vi "时间日期字符串转时间数组.vi"(11 "日期/时间字符串":string) -> (3 "时间数组":i32[](array[numeric]))   [LabVIEW 2016, in "TimingControl.lvlib" / "TimingControl.lvclass"]
uses:
  TimingControl.lvclass
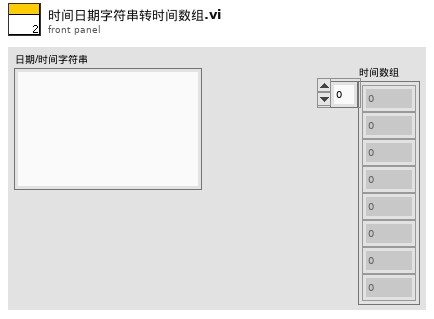
[diagram p1: front panel]
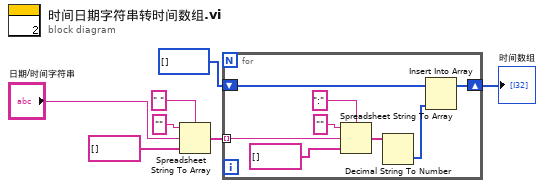
[diagram p0: block diagram]
diagram:
  n1 = Spreadsheet String To Array(delimiter (Tab)=" " ("分隔符(Tab)"), format string="" ("格式字符串"), spreadsheet string="日期/时间字符串", array type (2D Dbl)=string[] []) -> (array=w3:string[])
  n2 = for {
    tunnel: w3 -> [w13] mode=indexing
    shift-right: [w10] -> w1
    shift-left: i32[] [] -> [w11]
    n3 = Spreadsheet String To Array(delimiter (Tab)=":" ("分隔符(Tab)"), format string="" ("格式字符串"), spreadsheet string=w13, array type (2D Dbl)=string[] []) -> (array=w9:string[])
    n4 = Decimal String To Number(string=w9) -> (number=w8:i32[])  [unwired: 2 in, 1 out]
    n5 = Insert Into Array(array=w11, new element=w8) -> (w10:i32[])  [unwired: 1 in]
  }
  "时间数组" <- w1
